vi "FPGA Acquire.vi"(0 "Logging queue in":T6, 1 "Max allowed trial length (sec)":dbl=15.0 format="%#_13g", 5 "Logging queue element":T1={"Imaging Protocol"=enum."Live Imaging", "Number of Trials"=0, "Frame Size"=512, "# Averaged frames"=0, "Dwell time (us)"=0.0, "Index of Z-plane"=0, "Timelapse?"=FALSE, "Logging process is active"=FALSE, "Speed logging enabled"=FALSE, "tdms file ref"=refnum, "path"=path "", "Trial Number"=0, "Expected # points acquired"=FALSE, "Manually stopped"=FALSE, "Last trial"=FALSE, "Ch0 data"=[], "Ch1 data"=[], "Image Time"=[], "Continuous Time"=[], "Points acquired"={"Ch0 last trial"=0, "Ch1 last trial"=0, "All trials"=0}, "HW Timings File"=refnum} {"Frame Size" items=["100X100"=100, "128X128"=128, "200X200"=200, "256X256"=256, "512X512"=512, "1024x1024"=1024, "2048x2048"=2048]; "Dwell time (us)" format="%#.6g"}, 7 "FPGA Ref":T5, 9 "Target number of points":u64, 11 "error in (no error)":errorcluster, 13 "Imaging Protocol":T2) -> (4 "Logging queue out":T6, 6 "Logging queue element 2":T1={"Imaging Protocol"=enum."Live Imaging", "Number of Trials"=0, "Frame Size"=512, "# Averaged frames"=0, "Dwell time (us)"=0.0, "Index of Z-plane"=0, "Timelapse?"=FALSE, "Logging process is active"=FALSE, "Speed logging enabled"=FALSE, "tdms file ref"=refnum, "path"=path "", "Trial Number"=0, "Expected # points acquired"=FALSE, "Manually stopped"=FALSE, "Last trial"=FALSE, "Ch0 data"=[], "Ch1 data"=[], "Image Time"=[], "Continuous Time"=[], "Points acquired"={"Ch0 last trial"=0, "Ch1 last trial"=0, "All trials"=0}, "HW Timings File"=refnum} {"Frame Size" items=["100X100"=100, "128X128"=128, "200X200"=200, "256X256"=256, "512X512"=512, "1024x1024"=1024, "2048x2048"=2048]; "Dwell time (us)" format="%#.6g"}, 8 "Elements Remaining":u32, 10 "VI exec time":u32, 15 "error out":errorcluster)   [LabVIEW 2017]
uses:
  Typedefs/Logging queue element.ctl
  Typedefs/Data queue ref.ctl
  Typedefs/Imaging Protocols enum.ctl
  Typedefs/Frame Size.ctl
  Typedefs/Acquired points count.ctl
  RIG-SPECIFIC FILES/FPGA Refs/FPGA Ref.ctl
panel:
  out "Array":u32[](array[numeric])
  out "Ref Elements Remaining":u32
  out "# elements in queue":i32
  out "VI exec interval":u32
  out "Execution rate (Hz) 3":i32 format="Execution Rate: %.0f Hz"
  out "Execution rate (Hz)":i32 format="Execution Rate: %.0f Hz"
  out "Trial completed or \nImaging stopped":bool
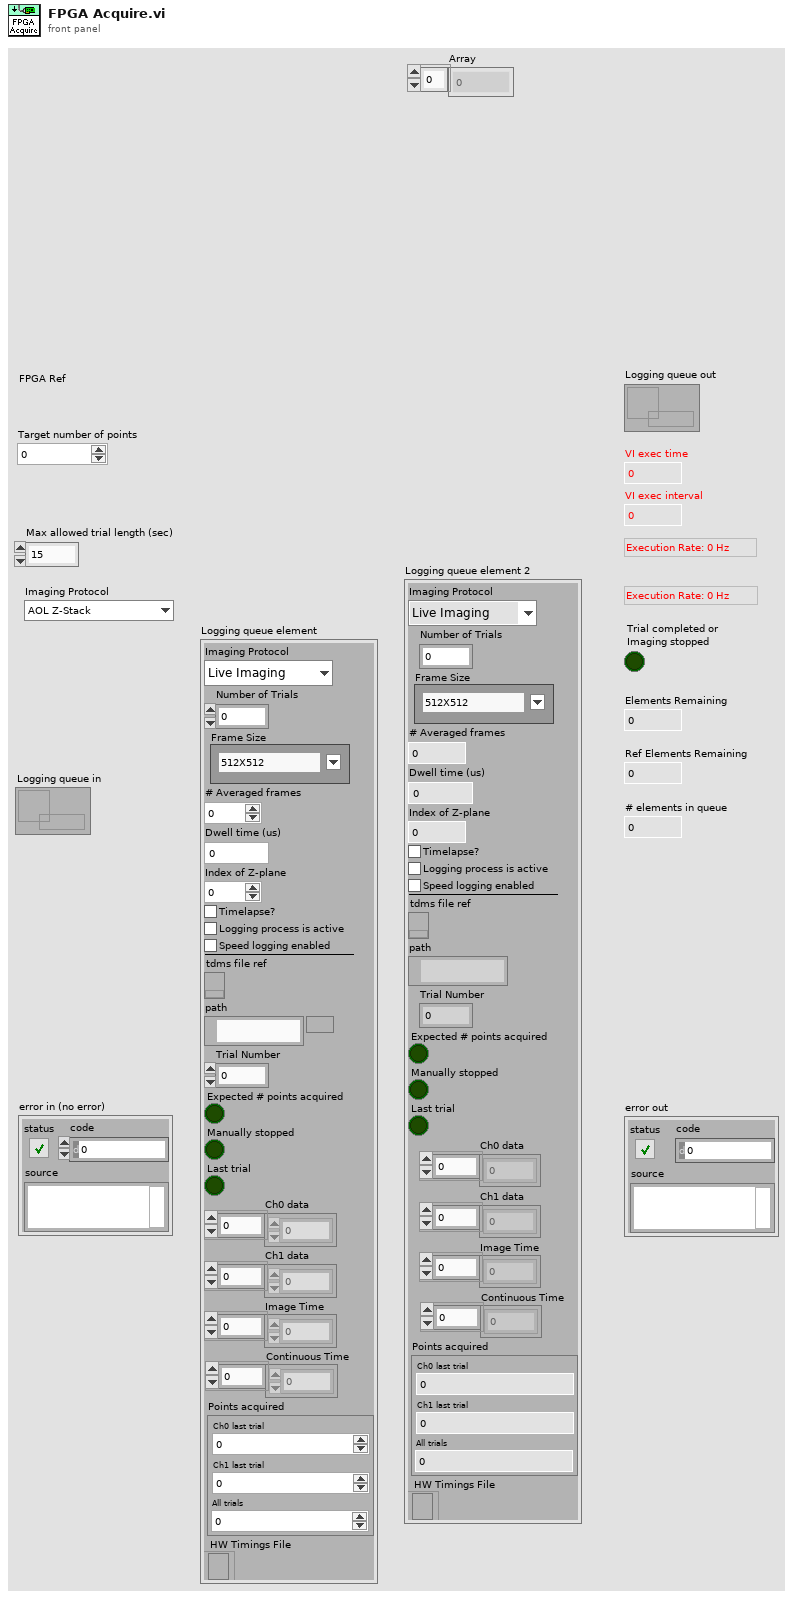
[diagram p1: front panel]
types:
  T1 = typedef "Logging queue element.ctl" = cluster{"Imaging Protocol":T2, "Number of Trials":u16, "Frame Size":T3, "# Averaged frames":u16, "Dwell time (us)":dbl, "Index of Z-plane":i32, "Timelapse?":bool, "Logging process is active":bool, "Speed logging enabled":bool, "tdms file ref":refnum<k34>, "path":path, "Trial Number":i32, "Expected # points acquired":bool, "Manually stopped":bool, "Last trial":bool, "Ch0 data":u32[], "Ch1 data":u32[], "Image Time":u64[], "Continuous Time":u64[], "Points acquired":T4, "HW Timings File":refnum<file>}
  T2 = typedef "Imaging Protocols enum.ctl" = enum16{"AOL Z-Stack", "Motor Z Stack", "Functional Acquisition", "Single Plane Acquisition", "Volume Acquisition", "Live Imaging", "Live Plane Imaging", "Live Volume Imaging"}
  T3 = typedef "Frame Size.ctl" = u16
  T4 = typedef "Acquired points count.ctl" = cluster{"Ch0 last trial":u64, "Ch1 last trial":u64, "All trials":u64}
  T5 = typedef "FPGA Ref.ctl" = refnum<k20>
  T6 = typedef "Data queue ref.ctl" = refnum<queue>
  T7 = typedef "FIFO elements available.ctl" = cluster{"Elements Available Ch0":u32, "Elements Available Ch1":u32, "Ref Elements Available":u32, "Ref Time Elements":u32, "Image Time Elements":u32, "Inter trial elements":u32}
  T8 = typedef "Logging queue element.ctl" = cluster{"Imaging Protocol":T2, "Number of Trials":u16, "Frame Size":T3, "# Averaged frames":u16, "Dwell time (us)":dbl, "Index of Z-plane":i32, "Timelapse?":bool, "Logging process is active":bool, "Speed logging enabled":bool, "tdms file ref":refnum<k34>, "path":path, "Trial Number":i32, "Expected # points acquired":bool, "Manually stopped":bool, "Last trial":bool, "Ch0 data":u32[], "Ch1 data":u32[], "Ref Data":u32[], "Ref Frame Time":u64[], "Image Time":u64[], "Continuous Time":u64[], "Ref X Length":u16, "Ref Y Length":u16, "# Ref Averaged frames":u16, "Ref Dwell time (us)":dbl, "Points acquired":T4, "HW Timings File":refnum<file>}
  T9 = typedef "Data arrays cluster.ctl" = cluster{"Ch0 data":u32[], "Ch1 data":u32[], "Ref data":u32[], "Ref time data":u64[], "Image time data":u64[], "Continuous time data":u64[]}
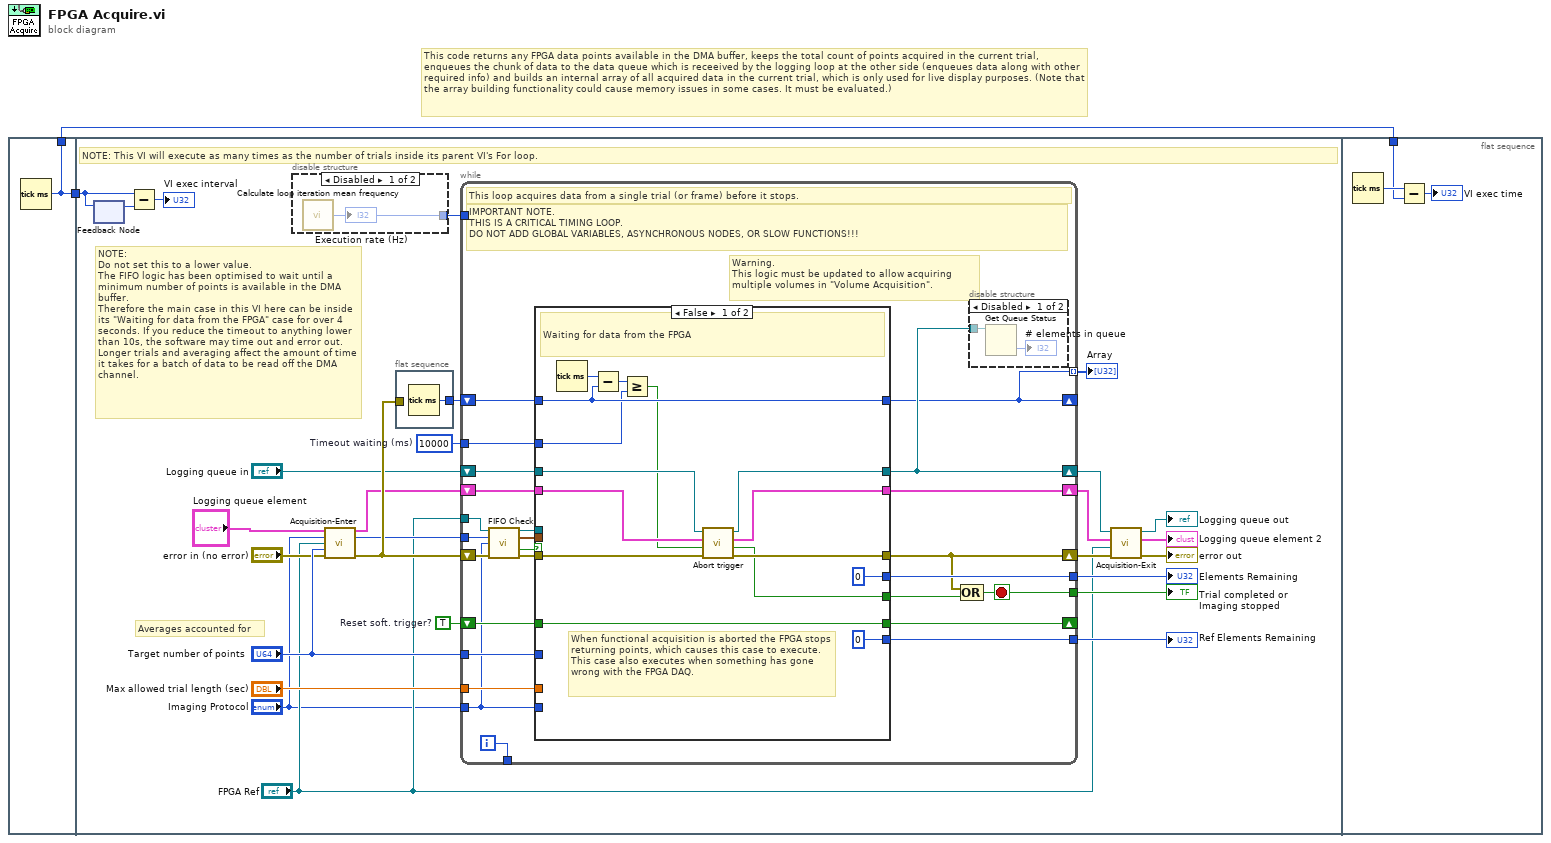
[diagram p0: block diagram]
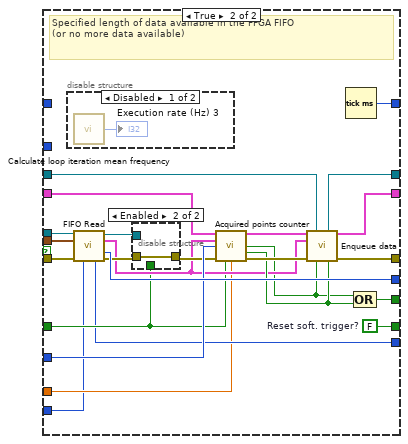
[diagram p4: hidden frame]
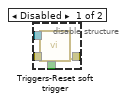
[diagram p5: hidden frame]
diagram:
  # "This code returns any FPGA data points available in the DMA buffer, keeps the total count of points acquired in the current trial, enqueues the chunk of data to the data queue which is receeived by the logging loop at the other side (enqueues data along with other required info) and builds an internal array of all acquired data in the current trial, which is only used for live display purposes. (Note that the array building functionality could cause memory issues in some cases. It must be evaluated.)"
  n1 = flat-sequence {
    tunnel: [w3] -> w1
    tunnel: [w3] -> w2
    tunnel: w2 -> [w20]
    tunnel: w1 -> [w106]
    frame #0 {
      n2 = Tick Count (ms)() -> (millisecond timer value=w3:u32)
    }
    frame #1 {
      w19 = TRUE  # Reset soft. trigger?
      w24 = u32 10000  # Timeout waiting (ms)
      # "NOTE:\nDo not set this to a lower value.\nThe FIFO logic has been optimised to wait until a minimum number of points is available in the DMA buffer.\nTherefore the main case in this VI here can be inside its \"Waiting for data from the FPGA\" case for over 4 seconds. If you reduce the timeout to anything lower than 10s, the software may time out and error out.\nLonger trials and averaging affect the amount of time it takes for a batch of data to be read off the DMA channel."
      # "Averages accounted for"
      # "NOTE: This VI will execute as many times as the number of trials inside its parent VI's For loop."
      n3 = feedback #1() -> (w22:u32)  [unwired: 1 in]
      n4 = feedback-in #1(w20) -> ()
      n5 = Subtract(x=w20, y=w22) -> (x-y=→"VI exec interval":u32)
      n6 = disable-structure shown="Disabled" {
        disable-tunnel: [w32 _] -> w23
        frame Disabled {
          n7 = call "Calculate loop iteration mean frequency.vi"() -> ("Refresh rate (Hz)"=w32:i32)  [unwired: 1 in]
          "Execution rate (Hz)" <- w32
        }
        frame Enabled {
        }
      }
      n8 = call "Acquisition-Enter.vi"("Logging queue element"="Logging queue element", "Imaging Protocol"="Imaging Protocol", "FPGA Ref"="FPGA Ref", "Target number of points"="Target number of points", "error in (no error)"="error in (no error)") -> ("Logging queue element"=w13:T1, "Read at least # points"=w18:u32, "error out"=w30:errorcluster)  [unwired: 8 in]
      n9 = flat-sequence {
        tunnel: [w31] -> w25
        tunnel: w30 -> [_]
        frame #0 {
          n10 = Tick Count (ms)() -> (millisecond timer value=w31:u32)
        }
      }
      n11 = while {
        tunnel: [w40] -> w12
        tunnel: [w53] -> w28
        shift-right: [w46] -> w9
        shift-left: "Logging queue in" -> [w54]
        shift-right: [w38] -> w26
        shift-left: w30 -> [w57]
        tunnel: "FPGA Ref" -> [w51]
        tunnel: w23 -> [_]
        shift-right: [w33] -> _
        shift-left: w25 -> [w50]
        tunnel: w24 -> [w49]
        shift-right: [w47] -> _
        shift-left: w19 -> [w48]
        tunnel: "Target number of points" -> [w44]
        tunnel: w18 -> [w43]
        tunnel: [w42] -> w17
        tunnel: "Max allowed trial length (sec)" -> [w41]
        shift-right: [w37] -> w10
        shift-left: w13 -> [w52]
        tunnel: [w36] -> _
        tunnel: "Imaging Protocol" -> [w34]
        tunnel: [w33] -> w5 mode=indexing
        i -> [w36]
        stop <- w40 stop-if-true
        # "IMPORTANT NOTE.\nTHIS IS A CRITICAL TIMING LOOP.\nDO NOT ADD GLOBAL VARIABLES, ASYNCHRONOUS NODES, OR SLOW FUNCTIONS!!!"
        # "Warning.\nThis logic must be updated to allow acquiring multiple volumes in \"Volume Acquisition\"."
        # "This loop acquires data from a single trial (or frame) before it stops."
        n12 = call "FIFO Check.vi"("FPGA Ref in"=w51, "Read at least # points"=w43, "Imaging Protocol"=w34, "error in (no error)"=w57) -> ("FPGA Ref out"=w56:T5, "Elements Available"=w35:T7, "Data available or data has just completed (read the FIFO)"=w45:bool, "error out"=w55:errorcluster)  [unwired: 7 in, 1 out]
        n13 = case shown="False" w45 {
          tunnel: w55 -> [w68 w94]
          tunnel: w56 -> [_ w96]
          tunnel: [w60 w89] -> w39
          tunnel: w44 -> [_ w91]
          tunnel: w52 -> [w62 w82]
          tunnel: w54 -> [w66 w81]
          tunnel: [w65 w80] -> w46
          tunnel: [w69 w90] -> w38
          tunnel: [u32 0 ("Elements Remaining") w99] -> w53
          tunnel: [w64 w78] -> w37
          tunnel: w50 -> [w71 _]
          tunnel: [w71 w97] -> w33
          tunnel: w49 -> [w70 _]
          tunnel: w48 -> [w67 w85]
          tunnel: [w67 w95] -> w47
          tunnel: [u32 0 ("Ref Elements Remaining") w84] -> w42
          tunnel: w41 -> [_ w83]
          tunnel: w35 -> [_ w77]
          tunnel: w34 -> [_ w76]
          frame False {
            # "When functional acquisition is aborted the FPGA stops returning points, which causes this case to execute. This case also executes when something has gone wrong with the FPGA DAQ."
            # "Waiting for data from the FPGA"
            n14 = Tick Count (ms)() -> (millisecond timer value=w72:u32)
            n15 = Subtract(x=w72, y=w71) -> (x-y=w73:u32)
            n16 = Greater Or Equal?(x=w73, y=w70) -> (x >= y?=w61:bool)
            n17 = call "Abort trigger.vi"("error in (no error)"=w68, "Timed out waiting on data"=w61, "Logging queue element in"=w62, "Logging queue in"=w66) -> ("error out"=w69:errorcluster, "Stop the acquisition module"=w60:bool, "Logging queue metadata shift out"=w64:T8, "Logging queue out"=w65:T6)  [unwired: 4 in]
          }
          frame True {
            w95 = FALSE  # Reset soft. trigger?
            # "Specified length of data available in the FPGA FIFO\n(or no more data available)"
            n18 = disable-structure shown="Disabled" {
              frame Disabled {
                n19 = call "Calculate loop iteration mean frequency.vi"() -> ("Refresh rate (Hz)"=→"Execution rate (Hz) 3":i32)  [unwired: 1 in]
              }
              frame Enabled {
              }
            }
            n20 = call "FIFO Read.vi"("FPGA Ref"=w96, "Elements Available"=w77, "error in"=w94, "Imaging Protocol"=w76) -> ("FPGA VI Reference Out"=w92:T5, "Data arrays cluster"=w86:T9, "Elements Remaining (Ch0)"=w99:u32, "Image Time Elements Remaining"=w84:u32, "error out"=w93:errorcluster)  [unwired: 7 in]
            n21 = disable-structure shown="Enabled" {
              disable-tunnel: w93 -> [w103 w104]
              disable-tunnel: w92 -> [w102 _]
              disable-tunnel: [w101 w104] -> w87
              disable-tunnel: w85 -> [w100 _]
              frame Disabled {
                n22 = call "Triggers-Reset soft trigger.vi"("Reset soft. trigger"=w100, "error in (no error)"=w103, "FPGA Ref"=w102) -> ("error out"=w101:errorcluster)  [unwired: 8 in]
              }
              frame Enabled {
              }
            }
            n23 = call "Acquired points counter.vi"("Logging queue element"=w82, "Raw Data Array"=w86, "Number of samples to be acquired (points in frame x Ch. x Av.)"=w91, "error in"=w87, "Initial reset"=w85, "Max allowed trial length (sec)"=w83) -> ("Logging queue element"=w79:T1, "Expected number of funct.acq points acquired on both channels"=w75:bool, "Live imaging stopped"=w88:bool, "error out"=w98:errorcluster)  [unwired: 6 in]
            n24 = call "Enqueue data.vi"("Logging queue element"=w79, "Logging queue in"=w81, "Chunk of data"=w86, "Error in"=w98, "Expected # points acquired"=w75, "Manually stopped"=w88) -> ("Logging queue out"=w80:T6, "Logging queue element"=w78:T1, "error out"=w90:errorcluster)  [unwired: 7 in]
            n25 = Tick Count (ms)() -> (millisecond timer value=w97:u32)
            n26 = Compound Arithmetic op=OR(w75, w88) -> (w89:bool)
          }
        }
        n27 = Compound Arithmetic op=OR(w38, w39) -> (w40:bool)
        n28 = disable-structure shown="Disabled" {
          disable-tunnel: w46 -> [w59 _]
          frame Disabled {
            n29 = Get Queue Status(queue=w59) -> (# elements in queue=→"# elements in queue":i32)  [unwired: 2 in, 7 out]
          }
          frame Enabled {
          }
        }
      }
      "Elements Remaining" <- w28
      "Trial completed or \nImaging stopped" <- w12
      "Ref Elements Remaining" <- w17
      "Array" <- w5
      n30 = call "Acquisition-Exit.vi"("error in (no error)"=w26, "FPGA Ref"="FPGA Ref", "Logging queue element"=w10, "Logging queue in"=w9) -> ("error out"=→"error out":errorcluster, "Logging queue element"=→"Logging queue element 2":T1, "Logging queue out"=→"Logging queue out":T6)  [unwired: 5 in]
    }
    frame #2 {
      n31 = Tick Count (ms)() -> (millisecond timer value=w107:u32)
      n32 = Subtract(x=w107, y=w106) -> (x-y=→"VI exec time":u32)
    }
  }
